vi "Tolerance_Check.vi"(0 "Top_Thresh":dbl, 1 "Tolerance":dbl, 2 "Input":dbl, 3 "Bottom_Thresh":dbl) -> (4 "Distance_from_unadjusted_top":dbl, 5 "Distance_from_unadjusted_bottom":dbl, 6 "Distance_from_adjusted_top":dbl, 7 "In_unadjusted_thresh":bool, 8 "In_adjusted_thresh":bool, 9 "Distance_from_adjusted_bottom":dbl)   [LabVIEW 2015]
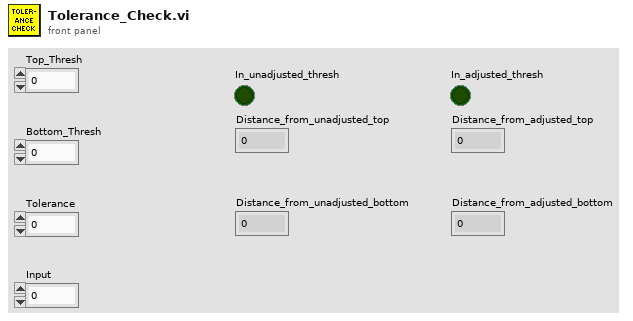
[diagram p1: front panel]
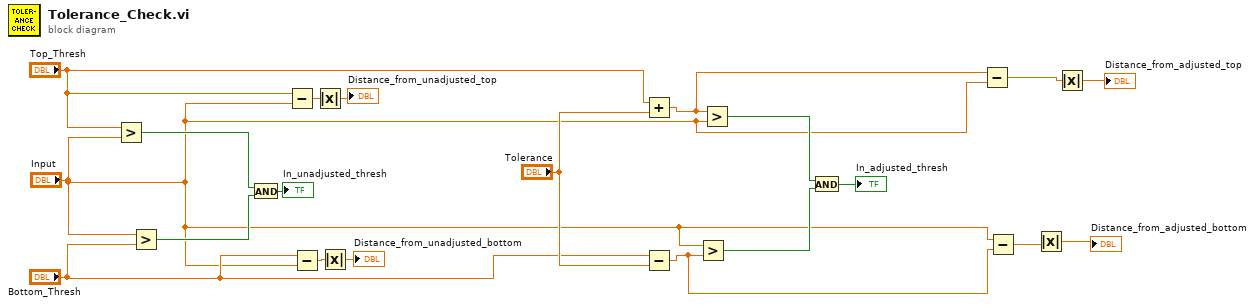
[diagram p0: block diagram]
diagram:
  n1 = Greater?(x="Top_Thresh", y="Input") -> (0:w20:bool)
  n2 = Greater?(x="Input", y="Bottom_Thresh") -> (0:w19:bool)
  n3 = And(x=w20, y=w19) -> (x .and. y?=→"In_unadjusted_thresh":bool)
  n4 = Subtract(x="Top_Thresh", y="Input") -> (x-y=w4:dbl)
  n5 = Subtract(x="Bottom_Thresh", y="Input") -> (x-y=w2:dbl)
  n6 = Absolute Value(x=w4) -> (abs(x)=→"Distance_from_unadjusted_top":dbl)
  n7 = Absolute Value(x=w2) -> (abs(x)=→"Distance_from_unadjusted_bottom":dbl)
  n8 = Add(x="Top_Thresh", y="Tolerance") -> (x+y=w11:dbl)
  n9 = Subtract(x="Bottom_Thresh", y="Tolerance") -> (x-y=w10:dbl)
  n10 = Greater?(x="Input", y=w10) -> (0:w12:bool)
  n11 = Greater?(x=w11, y="Input") -> (0:w13:bool)
  n12 = And(x=w13, y=w12) -> (x .and. y?=→"In_adjusted_thresh":bool)
  n13 = Subtract(x=w11, y="Input") -> (x-y=w7:dbl)
  n14 = Subtract(x="Input", y=w10) -> (x-y=w5:dbl)
  n15 = Absolute Value(x=w5) -> (abs(x)=→"Distance_from_adjusted_bottom":dbl)
  n16 = Absolute Value(x=w7) -> (abs(x)=→"Distance_from_adjusted_top":dbl)
